vi "Fake Actuator Measurements.vi"() -> (4 "Measurements":T6, 10 "Commands":T1, 15 "Within Limits":T5)   [LabVIEW 2009]
uses:
  Limits/Actuator Faults.ctl
  Limits/Cart Force Faults.ctl
  Limits/Cart Disp Faults.ctl
  Act & Cart Commands.ctl
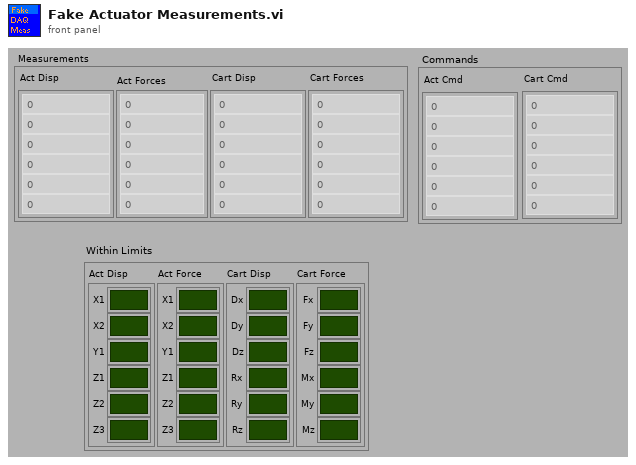
[diagram p1: front panel]
types:
  T1 = typedef "Act & Cart Commands.ctl" = cluster{"Act Cmd":dbl[], "Cart Cmd":dbl[]}
  T2 = typedef "Actuator Faults.ctl" = cluster{"X1":bool, "X2":bool, "Y1":bool, "Z1":bool, "Z2":bool, "Z3":bool}
  T3 = typedef "Cart Force Faults.ctl" = cluster{"Fx":bool, "Fy":bool, "Fz":bool, "Mx":bool, "My":bool, "Mz":bool}
  T4 = typedef "Cart Disp Faults.ctl" = cluster{"Dx":bool, "Dy":bool, "Dz":bool, "Rx":bool, "Ry":bool, "Rz":bool}
  T5 = cluster{"Act Disp":T2, "Act Force":T2, "Cart Force":T3, "Cart Disp":T4}
  T6 = cluster{"Act Disp":dbl[], "Act Forces":dbl[], "Cart Disp":dbl[], "Cart Forces":dbl[]}
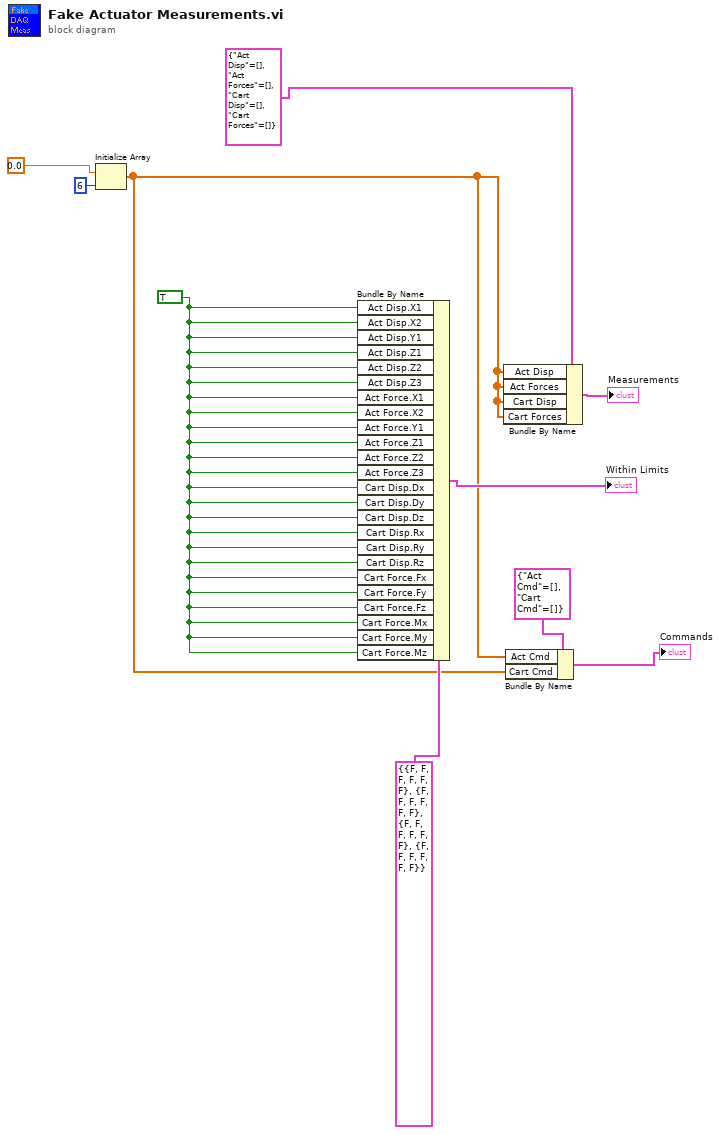
[diagram p0: block diagram]
diagram:
  w4 = TRUE ("Act Disp.X1")
  n1 = Initialize Array(0.0, 6 ("dimension size")) -> (w1:dbl[])
  n2 = Bundle By Name(cluster=T5 {"Act Disp"={"X1"=FALSE, "X2"=FALSE, "Y1"=FALSE, "Z1"=FALSE, "Z2"=FALSE, "Z3"=FALSE}, "Act Force"={"X1"=FALSE, "X2"=FALSE, "Y1"=FALSE, "Z1"=FALSE, "Z2"=FALSE, "Z3"=FALSE}, "Cart Force"={"Fx"=FALSE, "Fy"=FALSE, "Fz"=FALSE, "Mx"=FALSE, "My"=FALSE, "Mz"=FALSE}, "Cart Disp"={"Dx"=FALSE, "Dy"=FALSE, "Dz"=FALSE, "Rx"=FALSE, "Ry"=FALSE, "Rz"=FALSE}} ("Faults"), "Act Disp.X1"=w4, "Act Disp.X2"=w4, "Act Disp.Y1"=w4, "Act Disp.Z1"=w4, "Act Disp.Z2"=w4, "Act Disp.Z3"=w4, "Act Force.X1"=w4, "Act Force.X2"=w4, "Act Force.Y1"=w4, "Act Force.Z1"=w4, "Act Force.Z2"=w4, "Act Force.Z3"=w4, "Cart Disp.Dx"=w4, "Cart Disp.Dy"=w4, "Cart Disp.Dz"=w4, "Cart Disp.Rx"=w4, "Cart Disp.Ry"=w4, "Cart Disp.Rz"=w4, "Cart Force.Fx"=w4, "Cart Force.Fy"=w4, "Cart Force.Fz"=w4, "Cart Force.Mx"=w4, "Cart Force.My"=w4, "Cart Force.Mz"=w4) -> (→"Within Limits":T5)
  n3 = Bundle By Name(cluster=T6 {"Act Disp"=[], "Act Forces"=[], "Cart Disp"=[], "Cart Forces"=[]} ("Actuator Measurements"), "Act Disp"=w1, "Act Forces"=w1, "Cart Disp"=w1, "Cart Forces"=w1) -> (→"Measurements":T6)
  n4 = Bundle By Name(cluster=T1 {"Act Cmd"=[], "Cart Cmd"=[]} ("Cartesian Commands"), "Act Cmd"=w1, "Cart Cmd"=w1) -> (→"Commands":T1)
